vi "Read TempData.vi"(8 "error in (no error)":errorcluster, 11 "SetTemp Message":refnum<class "SetTemp Message.lvclass">) -> (0 "error out":errorcluster, 2 "TempData":cluster{"Temp":dbl, "Humid":dbl}, 3 "SetTemp Message":refnum<class "SetTemp Message.lvclass">)   [LabVIEW 2018, in "QMH_Class.lvlib" / "TestManager.lvlib" / "SetTemp Message.lvclass"]
uses:
  SetTemp Message.lvclass
  SetTemp Message.lvclass/SetTemp Message.ctl
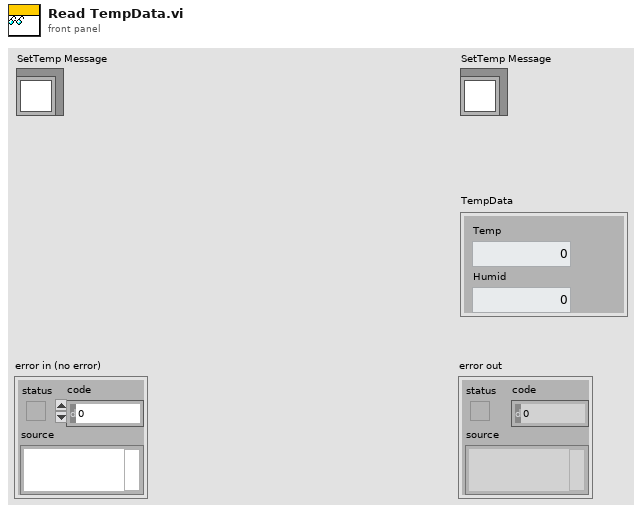
[diagram p1: front panel]
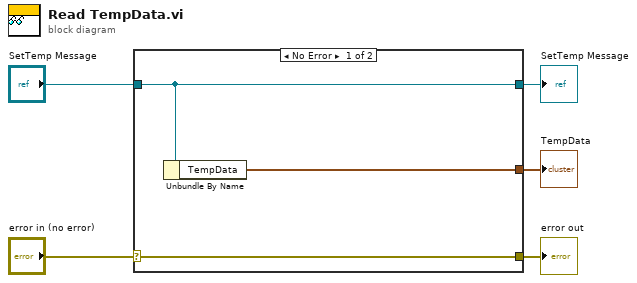
[diagram p0: block diagram]
diagram:
  n1 = case shown="No Error" "error in (no error)" {
    selector: "error in (no error)" -> [w8 w9]
    tunnel: [w8 w9] -> w4
    tunnel: [w7 w10] -> w2
    tunnel: "SetTemp Message" -> [w7 w10]
    tunnel: [w6 _] -> w1
    frame No Error {
      n2 = Unbundle By Name(w7) -> ("TempData"=w6:cluster{"Temp":dbl, "Humid":dbl})
    }
    frame Error {
    }
  }
  "error out" <- w4
  "SetTemp Message" <- w2
  "TempData" <- w1
